vi "EPR run.vi"(0 "control task in":refnum<k21>, 1 "sig task in":refnum<k21>, 2 "ref task in":refnum<k21>, 3 "error in":errorcluster, 4 "file path (dialog if empty)":path, 6 "Measurement Interval":dbl=1.0) -> ()   [LabVIEW 2012]
uses:
  <vilib>/DAQmx/read.llb/DAQmx Read (Counter U32 1Chan 1Samp).vi
  <vilib>/Utility/file.llb/Write To Spreadsheet File (I64).vi
  <vilib>/DAQmx/miscellaneous.llb/DAQmx Fill In Error Info.vi
panel:
  out "ref":u32
  in  "stop":bool
  out "signal":u32
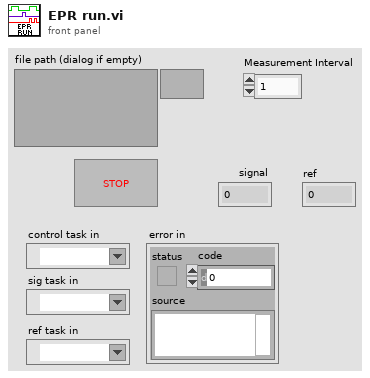
[diagram p1: front panel]
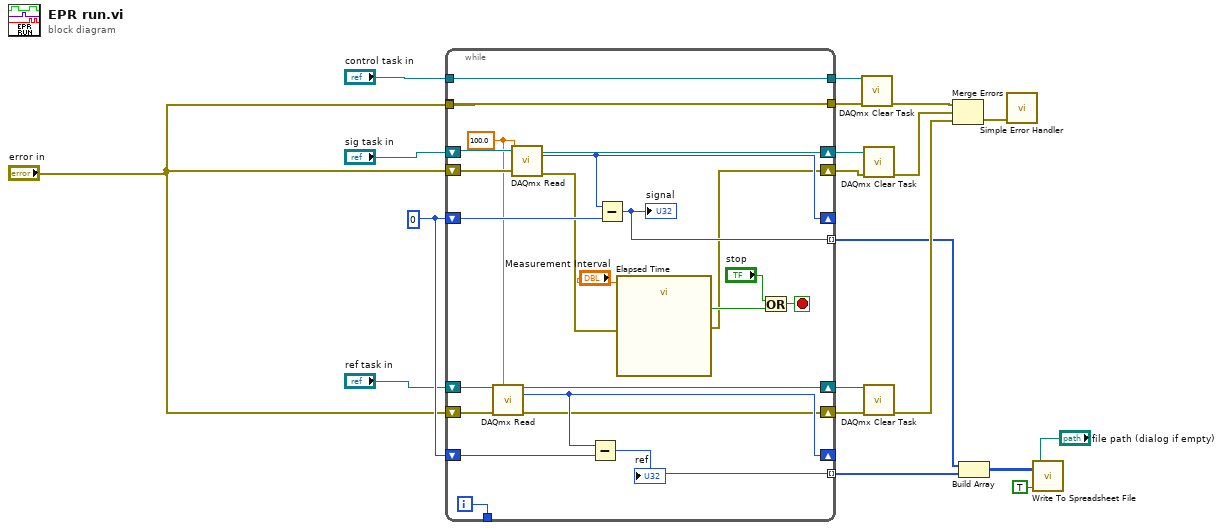
[diagram p0: block diagram]
diagram:
  w9 = u32 0 ("data")
  n1 = while {
    shift-right: [w33] -> w8
    shift-left: "sig task in" -> [w43]
    tunnel: [w36] -> w13 mode=indexing
    tunnel: "control task in" -> [w39]
    tunnel: [w23] -> _
    tunnel: [w39] -> w12
    tunnel: [w23] -> w11
    shift-right: [w29] -> _
    shift-left: w9 -> [w38]
    shift-right: [w30] -> _
    shift-left: w9 -> [w37]
    shift-right: [w31] -> w18
    shift-left: "ref task in" -> [w34]
    tunnel: [w28] -> w5 mode=indexing
    shift-right: [w27] -> w7
    shift-left: "error in" -> [w25]
    shift-right: [w26] -> w6
    shift-left: "error in" -> [w24]
    tunnel: "error in" -> [w23]
    tunnel: [w22] -> _
    i -> [w22]
    stop <- w42 stop-if-true
    w21 = 100.0 ("timeout")
    n2 = call-poly <vilib>:"DAQmx Read.vi"("task/channels in"=w34, "timeout"=w21, "error in"=w24) -> ("task out"=w31:refnum<k21>, "data"=w30:u32, "error out"=w26:errorcluster)  [unwired: 10 in]
    n3 = call-poly <vilib>:"DAQmx Read.vi"("task/channels in"=w43, "timeout"=w21, "error in"=w25) -> ("task out"=w33:refnum<k21>, "data"=w29:u32, "error out"=w32:errorcluster)  [unwired: 10 in]
    n4 = Subtract(x=w30, y=w37) -> (x-y=w36:u32)
    "ref" <- w36
    n5 = Subtract(x=w29, y=w38) -> (x-y=w28:u32)
    "signal" <- w28
    n6 = call "Elapsed Time"("Time Target (s)"="Measurement Interval", "error in (no error)"=w32) -> ("Time has Elapsed"=w41:bool, "error out"=w27:errorcluster)  [unwired: 10 in, 6 out]
    n7 = Or(x="stop", y=w41) -> (x .or. y?=w42:bool)
  }
  n8 = call <vilib>:"DAQmx Clear Task.vi"("task in"=w12, "error in"=w11) -> ("error out"=w10:errorcluster)  [unwired: 13 in]
  n9 = call <vilib>:"DAQmx Clear Task.vi"("task in"=w8, "error in"=w7) -> ("error out"=w16:errorcluster)  [unwired: 13 in]
  n10 = call <vilib>:"DAQmx Clear Task.vi"("task in"=w18, "error in"=w6) -> ("error out"=w14:errorcluster)  [unwired: 13 in]
  n11 = Merge Errors(w10, w16, w14) -> (w15:errorcluster)
  n12 = Build Array(w5, w13) -> (w17:u32[][])
  n13 = call <vilib>:"Simple Error Handler.vi"("error in (no error)"=w15) -> ()  [unwired: 4 in, 5 out]
  n14 = call-poly <vilib>:"Write To Spreadsheet File.vi"("transpose? (no:F)"=TRUE, "2D data"=w17, "file path (dialog if empty)"="file path (dialog if empty)") -> ()  [unwired: 5 in, 1 out]
